vi "Keyed Array Map String.vi"(0 "default":string, 1 "case matching (sensitive)":T1=enum."system", 4 "key":string, 5 "keys":string[](array[string]), 6 "values":string[](array[string])) -> (2 "index":i32, 3 "valid key":bool, 7 "value":string)   [LabVIEW 2020, in "NI_FTP.lvlib"]
uses:
  <vilib>/FTP/NI_FTP.lvlib
  <vilib>/FTP/util/Case Matching.ctl
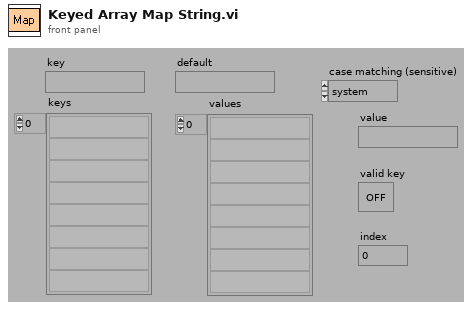
[diagram p1: front panel]
types:
  T1 = typedef "NI_FTP.lvlib/Case Matching.ctl" = enum16{"a != A", "a == A", "system"}
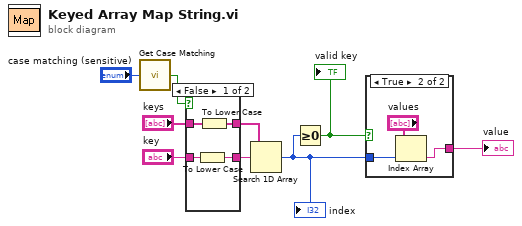
[diagram p0: block diagram]
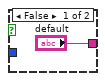
[diagram p3: hidden frame]
diagram:
  n1 = call <vilib>:"Get Case Matching.vi"("string matching"="case matching (sensitive)") -> ("match case"=w2:bool)
  n2 = case shown="False" w2 {
    tunnel: "keys" -> [w13 w15]
    tunnel: "key" -> [w11 w14]
    tunnel: [w12 w15] -> w4
    tunnel: [w10 w14] -> w3
    frame False {
      n3 = To Lower Case(string=w11) -> (all lower case string=w10:string)
      n4 = To Lower Case(string=w13) -> (all lower case string=w12:string[])
    }
    frame True {
    }
  }
  n5 = Search 1D Array(1D array=w4, element=w3) -> (index of element=w9:i32)  [unwired: 1 out]
  "index" <- w9
  n6 = Greater Or Equal To 0?(x=w9) -> (x >= 0?=w7:bool)
  "valid key" <- w7
  n7 = case shown="True" w7 {
    tunnel: ["default" w19] -> w8
    tunnel: w9 -> [_ w17]
    frame False {
    }
    frame True {
      n8 = Index Array(array="values", index=w17) -> (element=w19:string)
    }
  }
  "value" <- w8
